vi "主程序.vi"() -> ()   [LabVIEW 2010]
panel:
  out "SQRT":dbl
  in  "Number":dbl
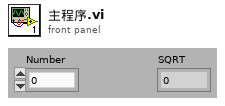
[diagram p1: front panel]
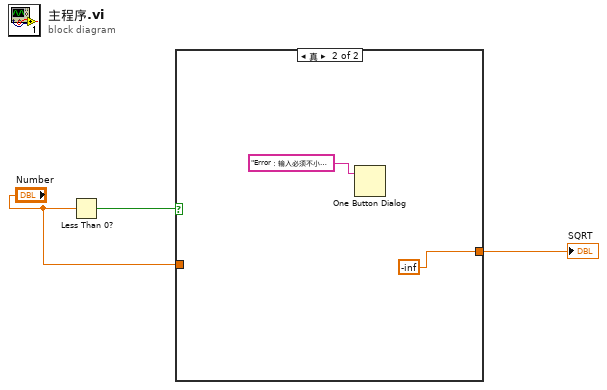
[diagram p0: block diagram]
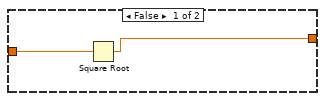
[diagram p2: hidden frame]
diagram:
  n1 = Less Than 0?(x="Number") -> (x < 0?=w3:bool)
  n2 = case shown="真" w3 {
    tunnel: "Number" -> [w5 _]
    tunnel: [w4 -inf] -> w1
    frame False {
      n3 = Square Root(x=w5) -> (sqrt(x)=w4:dbl)
    }
    frame True {
      n4 = One Button Dialog(message="Error：输入必须不小于0") -> ()  [unwired: 1 in, 1 out]
    }
  }
  "SQRT" <- w1
